vi "Untitled 5.vi"(8 "error in (no error)":errorcluster, 11 "Panel_UI in":refnum<class "Panel_UI.lvclass">) -> (0 "error out":errorcluster, 3 "Panel_UI out":refnum<class "Panel_UI.lvclass">)   [LabVIEW 2015, in "Panel_UI.lvclass"]
uses:
  Panel_UI.lvclass
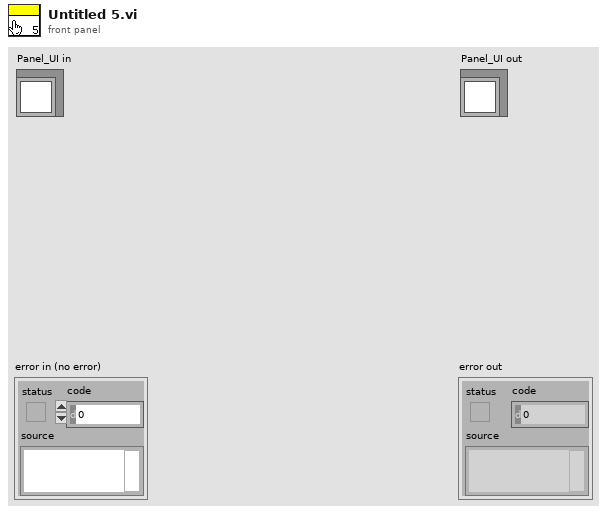
[diagram p1: front panel]
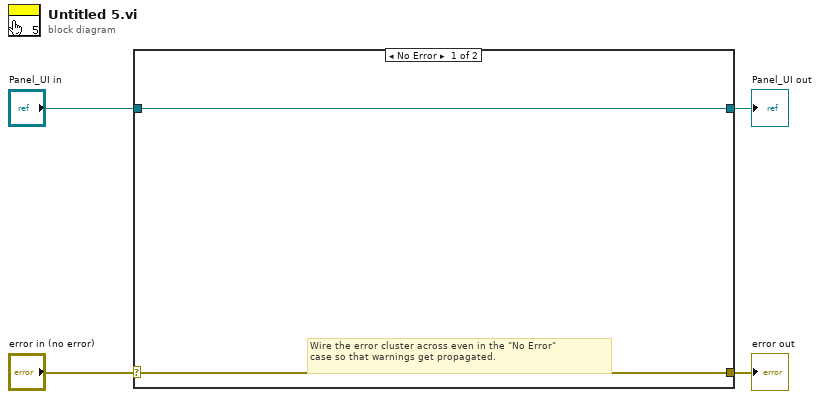
[diagram p0: block diagram]
diagram:
  n1 = case shown="No Error" "error in (no error)" {
    selector: "error in (no error)" -> [w5 w8]
    tunnel: [w5 w8] -> w3
    tunnel: [w6 w7] -> w1
    tunnel: "Panel_UI in" -> [w6 w7]
    frame No Error {
      # "Wire the error cluster across even in the \"No Error\"\ncase so that warnings get propagated."
    }
    frame Error {
    }
  }
  "error out" <- w3
  "Panel_UI out" <- w1
